vi "Print Console.vi"() -> ()   [LabVIEW 2009]
doc: "Cette console de file d'attente d'impression simule le contrôle des soumissions de travaux d'impression et surveille l'état des travaux d'impression en cours de traitement."
uses:
  Print Indicators.ctl
  Print Processing States.ctl
panel:
  out "Indicateurs d'impression":T1={"En attente"=TRUE, "Initialisation"=FALSE, "Impression"=FALSE, "Nombre de travaux"=0}
  out "Travaux d'impression\nen file d'attente":i32(slide) scale=0.0..25.0
  in  "Événement de file d'attente":bool
  in  "Stop":bool
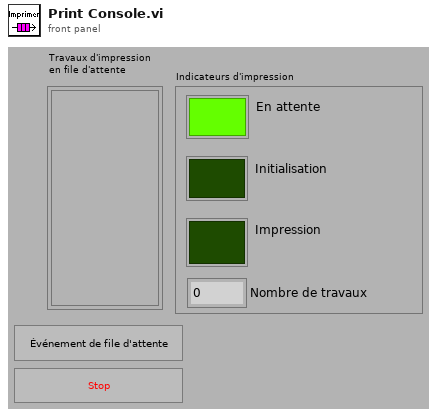
[diagram p1: front panel]
types:
  T1 = typedef "Print Indicators.ctl" = cluster{"En attente":bool, "Initialisation":bool, "Impression":bool, "Nombre de travaux":i32}
  T2 = typedef "Print Processing States.ctl" = enum16{"En attente", "Initialisation de la configuration", "Configuration", "Initialisation de l'impression", "Impression", "Arrêt"}
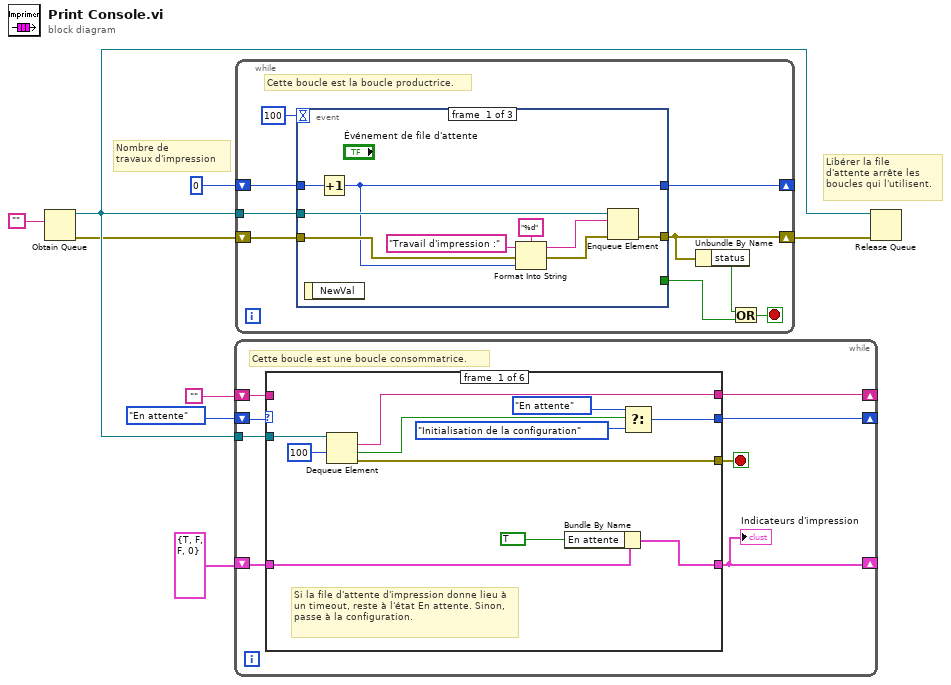
[diagram p0: block diagram]
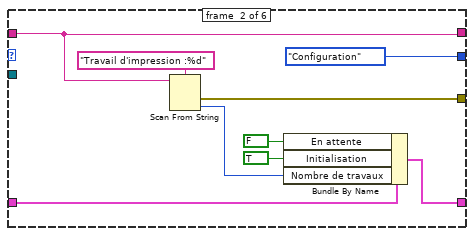
[diagram p2: hidden frame]
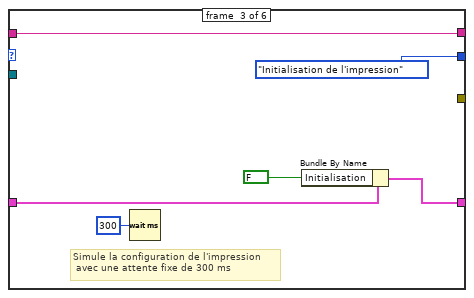
[diagram p3: hidden frame]
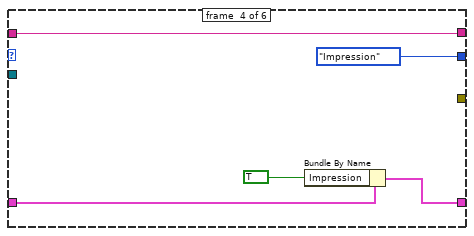
[diagram p4: hidden frame]
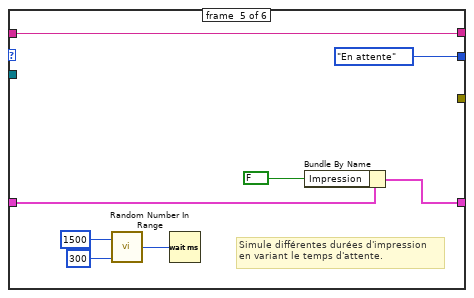
[diagram p5: hidden frame]
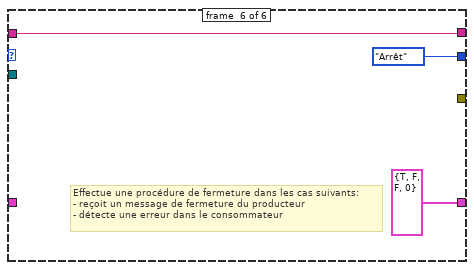
[diagram p6: hidden frame]
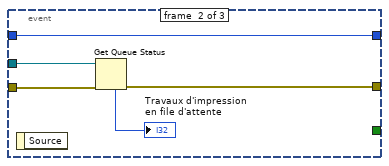
[diagram p7: hidden frame]
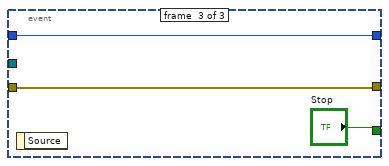
[diagram p8: hidden frame]
diagram:
  # "Nombre de\ntravaux d'impression"
  # "Libérer la file\nd'attente arrête les\nboucles qui l'utilisent."
  n1 = Obtain Queue ("Obtenir une file d'attente")(element data type="") -> (queue out=w7:refnum<queue>, error out=w1:errorcluster)  [unwired: 4 in, 1 out]
  n2 = while "Boucle While" {
    tunnel: w7 -> [w16]
    shift-right: [w10] -> _
    shift-left: Print_Processing_States."En attente" ("Enum") -> [w15]
    shift-right: [w13] -> _
    shift-left: T1 {"En attente"=TRUE, "Initialisation"=FALSE, "Impression"=FALSE, "Nombre de travaux"=0} ("Print LEDs") -> [w14]
    shift-right: [w11] -> _
    shift-left: "" -> [w12]
    stop <- w9 stop-if-true
    # "Cette boucle est une boucle consommatrice."
    n3 = case "Structure Condition" shown="\"Impression\"" w15 {
      tunnel: w16 -> [w27 _ _ _ _ _]
      tunnel: [w26 w28 _ _ _ _] -> w9
      tunnel: w14 -> [w21 w35 w41 w46 w54 _]
      tunnel: [w20 w34 w40 w45 w53 T1 {"En attente"=TRUE, "Initialisation"=FALSE, "Impression"=FALSE, "Nombre de travaux"=0} ("Print LEDs")] -> w13
      tunnel: [w18 Print_Processing_States."Configuration" ("Enum") Print_Processing_States."Initialisation de l'impression" ("Enum") Print_Processing_States."Impression" ("Enum") Print_Processing_States."En attente" ("Enum") Print_Processing_States."Arrêt" ("Enum")] -> w10
      tunnel: [w17 w31 w37 w43 w48 w56] -> w11
      tunnel: w12 -> [_ w31 w37 w43 w48 w56]
      frame #0 {
        # "Si la file d'attente d'impression donne lieu à un timeout, reste à l'état En attente. Sinon, passe à la configuration."
        n4 = Dequeue Element(queue=w27, timeout in ms (-1)=100) -> (element=w17:string, timed out?=w19:bool, error out=w26:errorcluster)  [unwired: 1 in, 1 out]
        n5 = Bundle By Name(cluster=w21, "En attente"=TRUE ("Waiting for\nnew job...")) -> (w20:T1)
        n6 = Select(t=Print_Processing_States."En attente" ("Enum"), s=w19, f=Print_Processing_States."Initialisation de la configuration" ("Enum")) -> (s? t:f=w18:T2)
      }
      frame #1 {
        n7 = Scan From String(format string="Travail d'impression :%d", input string=w31) -> (error out=w28:errorcluster, output 1=w29:i32)  [unwired: 3 in, 2 out]
        n8 = Bundle By Name(cluster=w35, "En attente"=FALSE ("Waiting for\nnew job..."), "Initialisation"=TRUE ("Waiting for\nnew job..."), "Nombre de travaux"=w29) -> (w34:T1)
      }
      frame #2 {
        # "Simule la configuration de l'impression\n avec une attente fixe de 300 ms"
        n9 = Wait (ms)(milliseconds to wait=u32 300) -> ()  [unwired: 1 out]
        n10 = Bundle By Name(cluster=w41, "Initialisation"=FALSE ("Waiting for\nnew job...")) -> (w40:T1)
      }
      frame #3 {
        n11 = Bundle By Name(cluster=w46, "Impression"=TRUE ("Waiting for\nnew job...")) -> (w45:T1)
      }
      frame #4 {
        # "Simule différentes durées d'impression\nen variant le temps d'attente."
        n12 = call "Random Number In Range.vi"("Limite inférieure"=u32 300 ("Lower Limit"), "Limite supérieure"=u32 1500 ("Upper Limit")) -> ("Nb aléatoire"=w49:u32)
        n13 = Wait (ms)(milliseconds to wait=w49) -> ()  [unwired: 1 out]
        n14 = Bundle By Name(cluster=w54, "Impression"=FALSE ("Waiting for\nnew job...")) -> (w53:T1)
      }
      frame #5 {
        # "Effectue une procédure de fermeture dans les cas suivants:\n- reçoit un message de fermeture du producteur\n- détecte une erreur dans le consommateur"
      }
    }
    "Indicateurs d'impression" <- w13
  }
  n15 = while "Boucle While" {
    tunnel: w7 -> [w67]
    shift-right: [w61] -> _
    shift-left: 0 -> [w62]
    shift-right: [w60] -> w2
    shift-left: w1 -> [w59]
    stop <- w65 stop-if-true
    # "Cette boucle est la boucle productrice."
    n16 = event "Structure Événement" shown="[1] Timeout" {
      selector: _ -> [_ _ _]
      dyn-events: _ -> [_ _ _]
      timeout: 100 -> [_ _ _]
      tunnel: w67 -> [w76 w79 _]
      tunnel: w59 -> [w74 w80 w82]
      tunnel: [w75 w78 w82] -> w60
      tunnel: [_ _ "Stop"] -> w66
      tunnel: w62 -> [w70 w77 w83]
      tunnel: [w68 w77 w83] -> w61
      event #0 {
        n17 = event-data() -> ()  [unwired: 1 in, 1 out]
        n18 = Increment(x=w70) -> (x+1=w68:i32)
        n19 = Format Into String(format string="%d", initial string="Travail d'impression :", error in=w74, w68) -> (resulting string=w69:string, error out=w73:errorcluster)
        n20 = Enqueue Element(queue=w76, element=w69, error in (no error)=w73) -> (error out=w75:errorcluster)  [unwired: 1 in, 2 out]
      }
      event #1 {
        n21 = event-data() -> ()  [unwired: 1 in, 1 out]
        n22 = Get Queue Status(queue=w79, error in (no error)=w80) -> (error out=w78:errorcluster, # elements in queue=→"Travaux d'impression\nen file d'attente":i32)  [unwired: 1 in, 6 out]
      }
      event #2 {
        n23 = event-data() -> ()  [unwired: 1 in, 1 out]
      }
    }
    n24 = Unbundle By Name ("Désassembler par nom")(w60) -> ("status"=w64:bool)
    n25 = Or ("OU")(x=w64, y=w66) -> (x .or. y?=w65:bool)
  }
  n26 = Release Queue ("Libérer une file d'attente")(queue=w7, error in (no error)=w2) -> ()  [unwired: 1 in, 3 out]
